vi "Alarms Create.vi"(8 "error in (no error)":errorcluster, 10 "Limits":T1, 11 "Alarms in":refnum<class "HK Alarms.lvclass">) -> (0 "error out":errorcluster, 3 "Alarms out":refnum<class "HK Alarms.lvclass">)   [LabVIEW 2024, in "HK Alarms.lvclass"]
uses:
  HK Alarms.lvclass
  HK Item/HK Channel Settings Limits.ctl
  HK Channel Settings Alarms.ctl
  HK Alarm enum Action.ctl
  HK Alarms.lvclass/HK Alarms.ctl
  HK Item/HK Item.lvclass
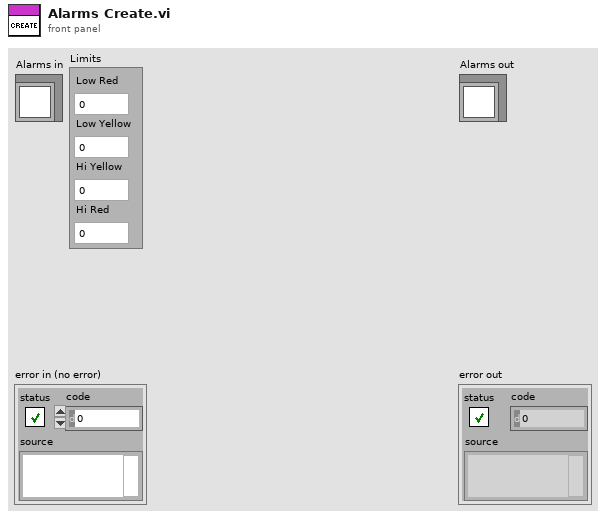
[diagram p1: front panel]
types:
  T1 = typedef "HK Item.lvclass/HK Channel Settings Limits.ctl" = cluster{"Low Red":dbl, "Low Yellow":dbl, "Hi Yellow":dbl, "Hi Red":dbl}
  T2 = typedef "HK Item.lvclass/HK Channel Settings Alarms.ctl" = cluster{"Enabled":bool, "Deadband":i32, "Action":T3}
  T3 = typedef "HK Item.lvclass/HK Alarm enum Action.ctl" = enum16{"Light", "Message", "Safe"}
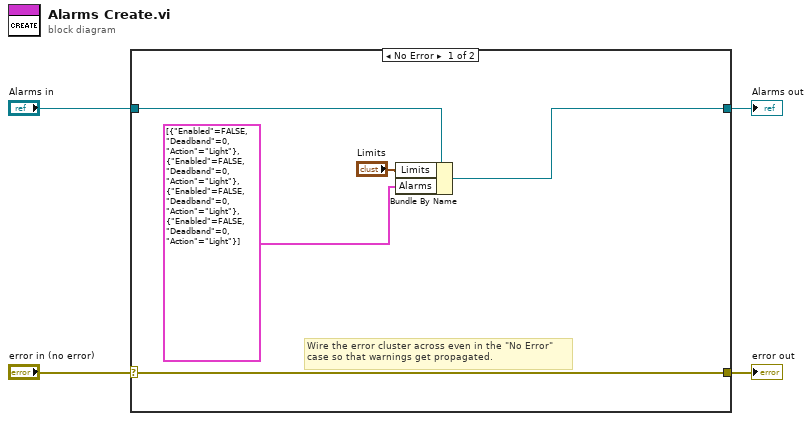
[diagram p0: block diagram]
diagram:
  n1 = case shown="No Error" "error in (no error)" {
    selector: "error in (no error)" -> [w9 w11]
    tunnel: [w9 w11] -> w3
    tunnel: [w7 w10] -> w1
    tunnel: "Alarms in" -> [w6 w10]
    frame No Error {
      # "Wire the error cluster across even in the \"No Error\"\ncase so that warnings get propagated."
      n2 = Bundle By Name(cluster=w6, "Limits"="Limits", "Alarms"=T2[] [{"Enabled"=FALSE, "Deadband"=0, "Action"=enum."Light"}, {"Enabled"=FALSE, "Deadband"=0, "Action"=enum."Light"}, {"Enabled"=FALSE, "Deadband"=0, "Action"=enum."Light"}, {"Enabled"=FALSE, "Deadband"=0, "Action"=enum."Light"}]) -> (w7:refnum<class "HK Alarms.lvclass">)
    }
    frame Error {
    }
  }
  "error out" <- w3
  "Alarms out" <- w1
